vi "cwlaserOpen.vi"   [LabVIEW 2017]
uses:
  globalDevices.vi
  <vilib>/Instr/_visa.llb/VISA Configure Serial Port (Instr).vi
types:
  T1 = cluster{"serialPort":refnum<visa-resource-name>, "error":errorcluster, "power (mW)":dbl, "wavelength (nm)":dbl, "type":string}[]
  T2 = cluster{"serialPort":refnum<visa-resource-name>, "error":errorcluster, "power (mW)":dbl, "wavelength (nm)":dbl, "type":string}
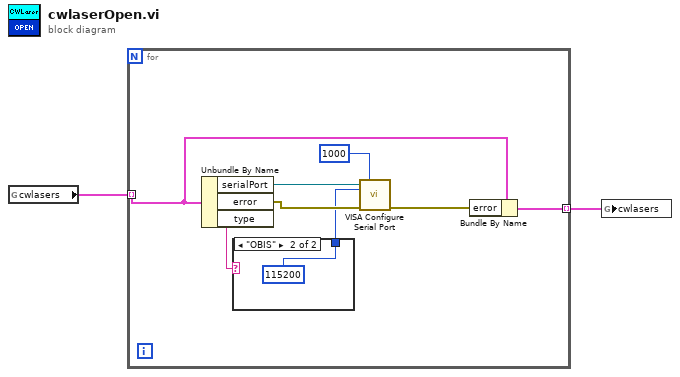
[diagram p0: block diagram]
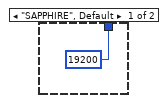
[diagram p2: hidden frame]
diagram:
  n1 = global read "globalDevices.vi" "cwlasers"() -> (w2:T1)
  n2 = for {
    tunnel: w2 -> [w8] mode=indexing
    tunnel: [w6] -> w1 mode=indexing
    n3 = Unbundle By Name(w8) -> ("serialPort"=w10:refnum<visa-resource-name>, "error"=w9:errorcluster, "type"=w4:string)
    n4 = case shown="\"OBIS\"" w4 {
      tunnel: [u32 19200 ("baud rate") u32 115200 ("baud rate")] -> w3
      frame "SAPPHIRE", Default {
      }
      frame "OBIS" {
      }
    }
    n5 = call-poly "VISA Configure Serial Port"("VISA resource name"=w10, "timeout (10sec)"=u32 1000, "baud rate (9600)"=w3, "error in (no error)"=w9) -> ("error out"=w7:errorcluster)  [unwired: 10 in, 1 out]
    n6 = Bundle By Name(cluster=w8, "error"=w7) -> (w6:T2)
  }
  n7 = global write "globalDevices.vi" "cwlasers"(w1) -> ()
